vi "Queue Manager.vi"(5 "Queue Name":T3, 6 "timeout in ms (-1)":i32=-1, 7 "Action":T2=enum."Enqueue", 8 "Error In":errorcluster, 11 "Message Packet Array":T1[](array[typedef])) -> (0 "Error Out":errorcluster, 1 "Empty?":bool, 3 "Message Packet [Out]":T1)   [LabVIEW 2014]
uses:
  Controls/QueueNames.ctl
  Controls/Queue Manager Actions.ctl
  Controls/MessagePacket.ctl
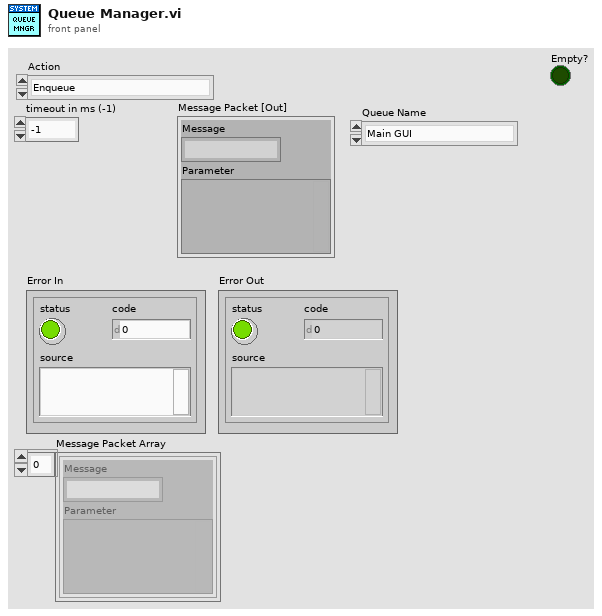
[diagram p1: front panel]
types:
  T1 = typedef "MessagePacket.ctl" = cluster{"Message":string, "Parameter":variant}
  T2 = typedef "Queue Manager Actions.ctl" = enum16{"Init", "Enqueue", "Enqueue All", "Preview Queue", "Dequeue", "Get Status", "Flush Queue", "Flush All Queues", "Release All Queues", "Release Queue", "Enqueue at Opposite End"}
  T3 = typedef "QueueNames.ctl" = enum16{"Main GUI", "Main Scan Processor", "Main Display", "Main Table Stage GUI", "Main Table Stage Proc.", "Scan Engine"}
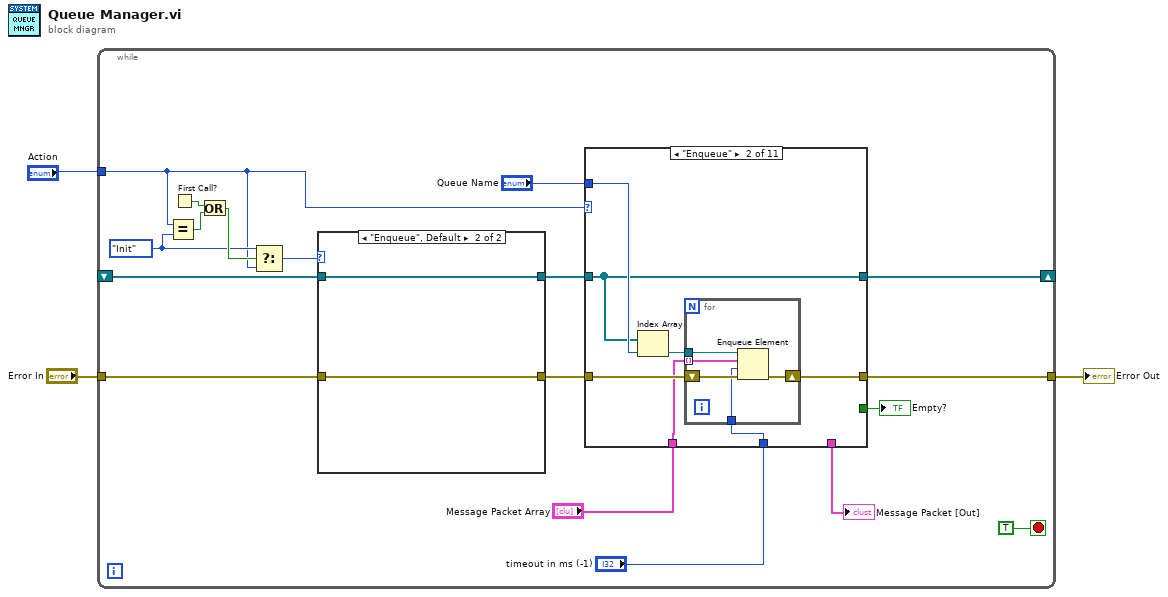
[diagram p0: block diagram]
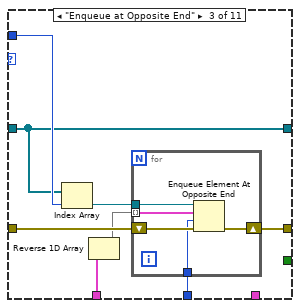
[diagram p3: hidden frame]
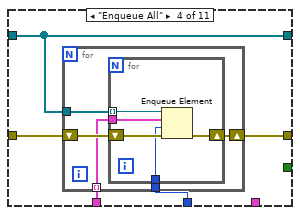
[diagram p4: hidden frame]
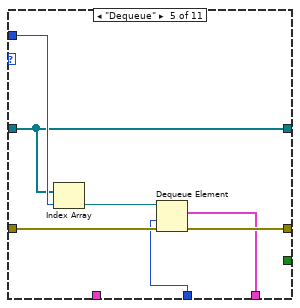
[diagram p5: hidden frame]
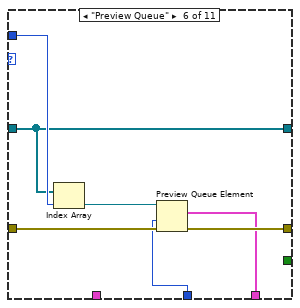
[diagram p6: hidden frame]
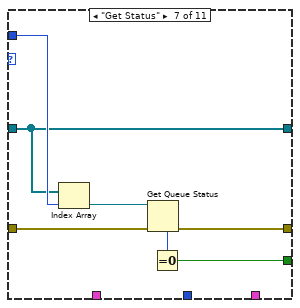
[diagram p7: hidden frame]
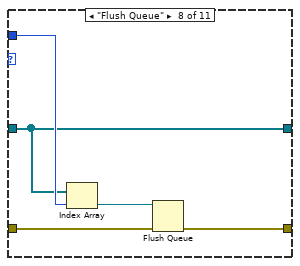
[diagram p8: hidden frame]
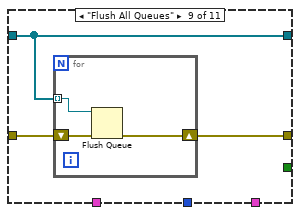
[diagram p9: hidden frame]
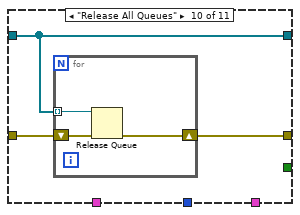
[diagram p10: hidden frame]
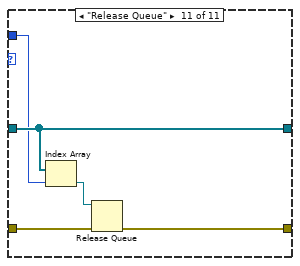
[diagram p11: hidden frame]
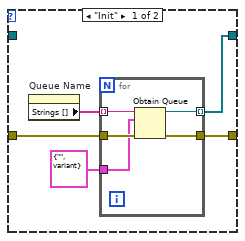
[diagram p12: hidden frame]
diagram:
  n1 = while {
    tunnel: "Action" -> [w5]
    tunnel: "Error In" -> [w16]
    tunnel: [w15] -> w1
    shift-right: [w7] -> _
    shift-left: _ -> [w6]
    stop <- TRUE stop-if-true
    w18 = Queue_Manager_Actions."Init"
    n2 = Equal?(x=w5, y=w18) -> (x = y?=w20:bool)
    n3 = First Call?() -> (First Call?: T/F=w21:bool)
    n4 = Or(x=w21, y=w20) -> (x .or. y?=w19:bool)
    n5 = Select(t=w18, s=w19, f=w5) -> (s? t:f=w17:T2)
    n6 = case shown="\"Enqueue\", Default" w17 {
      tunnel: [w110 w117] -> w12
      tunnel: w16 -> [w109 w118]
      tunnel: [w108 w118] -> w14
      tunnel: w6 -> [_ w117]
      frame "Init" {
        n7 = property on="Queue Name" class="Enum (strict)"() -> ("Strings []"=w111:string[])  [unwired: 2 in, 2 out]
        n8 = for {
          tunnel: w111 -> [w116] mode=indexing
          tunnel: [w115] -> w110 mode=indexing
          tunnel: w109 -> [w114]
          tunnel: [w113] -> w108
          tunnel: T1 {"Message"="", "Parameter"=variant} ("Message Packet") -> [w112]
          n9 = Obtain Queue(name (unnamed)=w116, element data type=w112, error in (no error)=w114) -> (queue out=w115:refnum<queue>, error out=w113:errorcluster)  [unwired: 2 in, 1 out]
        }
      }
      frame "Enqueue", Default {
      }
    }
    n10 = case shown="\"Enqueue\"" w5 {
      tunnel: w12 -> [w22 w25 w38 w50 w65 w72 w78 w85 w90 w96 w104]
      tunnel: [w23 w29 w42 w52 w69 w76 w83 w86 w91 w97 w105] -> w15
      tunnel: w14 -> [w23 w30 w43 w53 w70 w77 w84 w89 w92 w98 w106]
      tunnel: "Queue Name" -> [_ w28 w41 _ w68 w75 w82 w88 _ _ w103]
      tunnel: "Message Packet Array" -> [_ w26 w39 w51 _ _ _ _ _ _ _]
      tunnel: [_ _ _ _ w66 w73 _ _ _ _ _] -> w11
      tunnel: [_ _ _ _ _ _ w79 _ _ _ _] -> w10
      tunnel: [w22 w25 w38 w50 w65 w72 w78 w85 w90 w96 w104] -> w7
      tunnel: "timeout in ms (-1)" -> [_ w24 w36 w49 w64 w71 _ _ _ _ _]
      frame "Init", Default {
      }
      frame "Enqueue" {
        n11 = Index Array(array=w25, index=w28) -> (element=w27:refnum<queue>)
        n12 = for {
          tunnel: w27 -> [w33]
          tunnel: w26 -> [w32] mode=indexing
          shift-right: [w34] -> w29
          shift-left: w30 -> [w35]
          tunnel: w24 -> [w31]
          n13 = Enqueue Element(queue=w33, element=w32, timeout in ms (-1)=w31, error in (no error)=w35) -> (error out=w34:errorcluster)  [unwired: 2 out]
        }
      }
      frame "Enqueue at Opposite End" {
        n14 = Index Array(array=w38, index=w41) -> (element=w40:refnum<queue>)
        n15 = Reverse 1D Array(array=w39) -> (reversed array=w37:T1[])
        n16 = for {
          tunnel: w40 -> [w46]
          tunnel: w37 -> [w45] mode=indexing
          shift-right: [w47] -> w42
          shift-left: w43 -> [w48]
          tunnel: w36 -> [w44]
          n17 = Enqueue Element At Opposite End(queue=w46, element=w45, timeout in ms (-1)=w44, error in (no error)=w48) -> (error out=w47:errorcluster)  [unwired: 2 out]
        }
      }
      frame "Enqueue All" {
        n18 = for {
          tunnel: w51 -> [w56] mode=indexing
          shift-right: [w57] -> w52
          shift-left: w53 -> [w58]
          tunnel: w50 -> [w55]
          tunnel: w49 -> [w54]
          n19 = for {
            tunnel: w55 -> [w61] mode=indexing
            tunnel: w56 -> [w60]
            shift-right: [w62] -> w57
            shift-left: w58 -> [w63]
            tunnel: w54 -> [w59]
            n20 = Enqueue Element(queue=w61, element=w60, timeout in ms (-1)=w59, error in (no error)=w63) -> (error out=w62:errorcluster)  [unwired: 2 out]
          }
        }
      }
      frame "Dequeue" {
        n21 = Index Array(array=w65, index=w68) -> (element=w67:refnum<queue>)
        n22 = Dequeue Element(queue=w67, timeout in ms (-1)=w64, error in (no error)=w70) -> (element=w66:T1, error out=w69:errorcluster)  [unwired: 2 out]
      }
      frame "Preview Queue" {
        n23 = Index Array(array=w72, index=w75) -> (element=w74:refnum<queue>)
        n24 = Preview Queue Element(queue=w74, timeout in ms (-1)=w71, error in (no error)=w77) -> (element=w73:T1, error out=w76:errorcluster)  [unwired: 2 out]
      }
      frame "Get Status" {
        n25 = Index Array(array=w78, index=w82) -> (element=w81:refnum<queue>)
        n26 = Get Queue Status(queue=w81, error in (no error)=w84) -> (error out=w83:errorcluster, # elements in queue=w80:i32)  [unwired: 1 in, 6 out]
        n27 = Equal To 0?(x=w80) -> (x = 0?=w79:bool)
      }
      frame "Flush Queue" {
        n28 = Index Array(array=w85, index=w88) -> (element=w87:refnum<queue>)
        n29 = Flush Queue(queue=w87, error in (no error)=w89) -> (error out=w86:errorcluster)  [unwired: 2 out]
      }
      frame "Flush All Queues" {
        n30 = for {
          shift-right: [w94] -> w91
          shift-left: w92 -> [w95]
          tunnel: w90 -> [w93] mode=indexing
          n31 = Flush Queue(queue=w93, error in (no error)=w95) -> (error out=w94:errorcluster)  [unwired: 2 out]
        }
      }
      frame "Release All Queues" {
        n32 = for {
          shift-right: [w100] -> w97
          shift-left: w98 -> [w101]
          tunnel: w96 -> [w99] mode=indexing
          n33 = Release Queue(queue=w99, error in (no error)=w101) -> (error out=w100:errorcluster)  [unwired: 1 in, 2 out]
        }
      }
      frame "Release Queue" {
        n34 = Index Array(array=w104, index=w103) -> (element=w102:refnum<queue>)
        n35 = Release Queue(queue=w102, error in (no error)=w106) -> (error out=w105:errorcluster)  [unwired: 1 in, 2 out]
      }
    }
    "Message Packet [Out]" <- w11
    "Empty?" <- w10
  }
  "Error Out" <- w1
